vi "Get Ctr by Path.vi"() -> ()   [LabVIEW 2017]
uses:
  <vilib>/Utility/VariantDataType/VariantType.lvlib
panel:
  out "Value":variant
  out "Children":string
  in  "value":string="VI,127.0.0.1:3374,TC.vi/PNL_CTR,0/TAB_PAGE,0/PAGE_CTR,0/TAB_PAGE,10/PAGE_CTR,2"
  out "Cousins":string[](array[string])
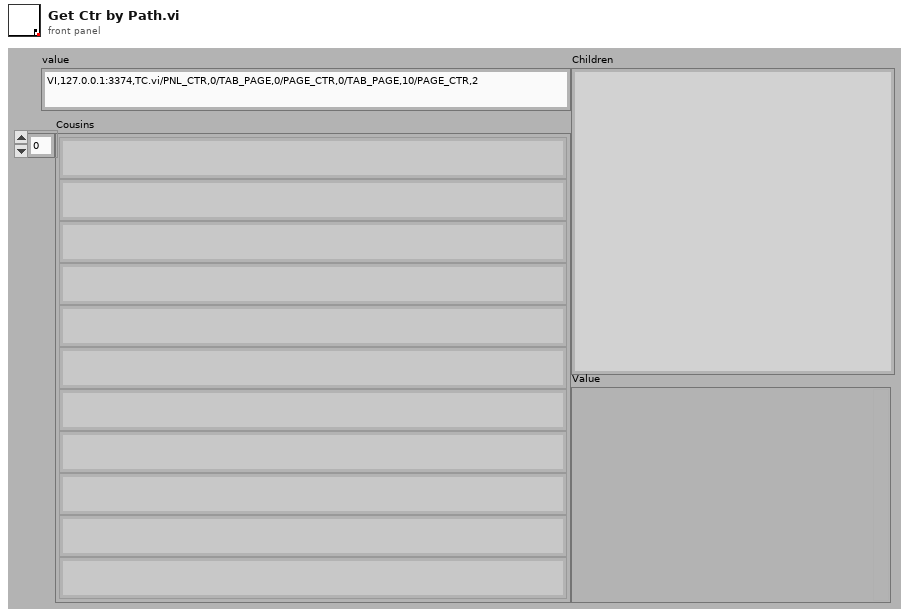
[diagram p1: front panel]
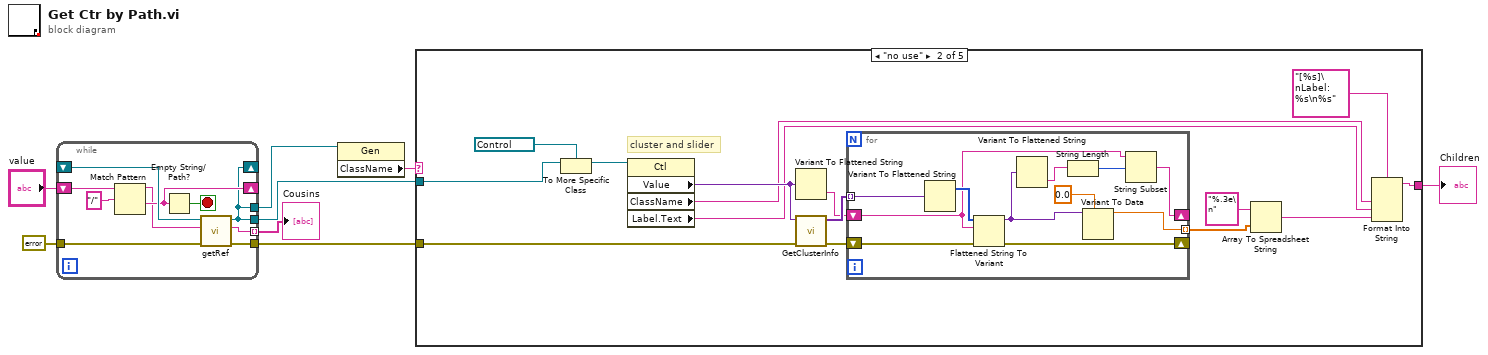
[diagram p0: block diagram]
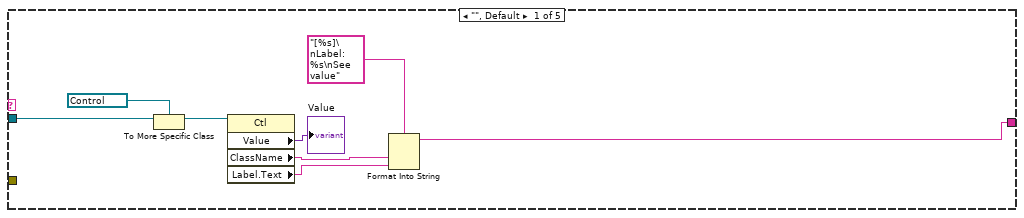
[diagram p2: hidden frame]
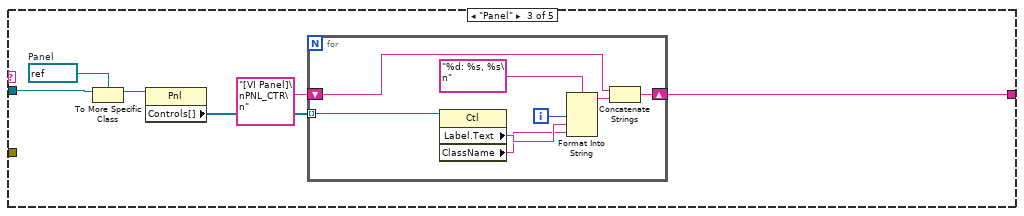
[diagram p3: hidden frame]
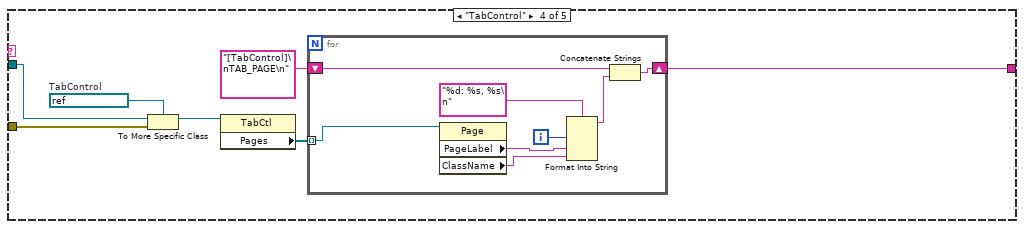
[diagram p4: hidden frame]
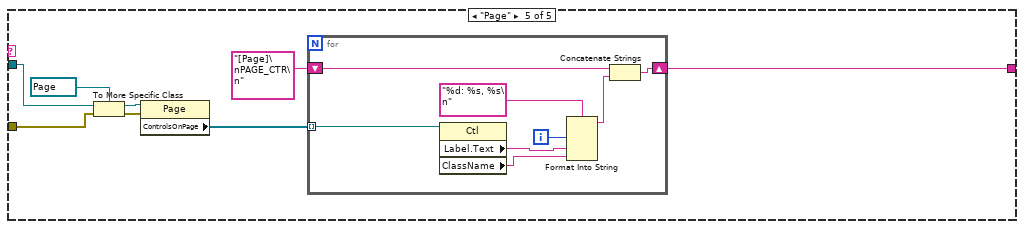
[diagram p5: hidden frame]
diagram:
  n1 = while {
    shift-right: [w14] -> _
    shift-left: "value" -> [w18]
    shift-right: [w9] -> _
    shift-left: _ -> [w15]
    tunnel: errorcluster {"status"=FALSE, "code"=0, "source"=""} ("error out") -> [w13]
    tunnel: [w12] -> w1
    tunnel: [w9] -> w8
    tunnel: [w10] -> w5 mode=indexing
    tunnel: [w9] -> w3
    stop <- w16 stop-if-true
    n2 = Match Pattern(string=w18, regular expression="/" ("搜索字符串/字符(-)")) -> (before substring=w11:string, after substring=w14:string)  [unwired: 3 out]
    n3 = Empty String/Path?(string/path=w14) -> (empty?=w16:bool)
    n4 = call "getRef.vi"("error in"=w13, "name"=w11, "Gen ref in"=w15) -> ("error out"=w12:errorcluster, "cousins"=w10:string, "Gen ref out"=w9:refnum<vi>)  [unwired: 6 out]
  }
  "Cousins" <- w5
  n5 = property class="Gen"(reference=w8) -> ("ClassName"=w4:string)  [unwired: 1 in, 2 out]
  n6 = case shown="\"no use\"" w4 {
    tunnel: w3 -> [w24 w39 w57 w72 w85]
    tunnel: [w22 w30 w53 w67 w82] -> w2
    tunnel: w1 -> [_ w37 _ w71 w86]
    frame "", Default {
      n7 = To More Specific Class(target class=refnum<vi> refnum ("引用"), reference=w24) -> (specific class reference=w26:refnum<vi>)  [unwired: 1 in, 1 out]
      n8 = property class="Ctl"(reference=w26) -> ("Value"=→"Value":variant, "ClassName"=w20:string, "Label.Text"=w19:string)  [unwired: 1 in, 2 out]
      n9 = Format Into String(format string="[%s]\nLabel: %s\nSee value", w20, w19) -> (resulting string=w22:string)  [unwired: 2 in, 1 out]
    }
    frame "no use" {
      # "cluster and slider"
      n10 = To More Specific Class(target class=refnum<vi> refnum ("引用"), reference=w39) -> (specific class reference=w41:refnum<vi>)  [unwired: 1 in, 1 out]
      n11 = property class="Ctl"(reference=w41) -> ("Value"=w38:variant, "ClassName"=w29:string, "Label.Text"=w28:string)  [unwired: 1 in, 2 out]
      n12 = Variant To Flattened String(Variant=w38) -> (data string=w35:string)  [unwired: 1 out]
      n13 = call <vilib>:"GetClusterInfo.vi"("error in (no error)"=w37, "Variant"=w38) -> ("error out"=w34:errorcluster, "Cluster Elements"=w36:variant[])  [unwired: 8 out]
      n14 = for {
        tunnel: w36 -> [w52] mode=indexing
        shift-right: [w47] -> _
        shift-left: w35 -> [w48]
        shift-right: [w45] -> _
        shift-left: w34 -> [w46]
        tunnel: [w42] -> w33 mode=indexing
        n15 = Variant To Flattened String(Variant=w52) -> (1:w51:i16[])  [unwired: 1 out]
        n16 = Flattened String To Variant(4:w46, 6:w48, 7:w51) -> (0:w45:errorcluster, 3:w44:variant)
        n17 = Variant To Flattened String(Variant=w44) -> (data string=w50:string)  [unwired: 1 out]
        n18 = String Length(string=w50) -> (length=w49:i32)
        n19 = Variant To Data(type=0.0, Variant=w44) -> (data=w42:dbl)  [unwired: 1 in, 1 out]
        n20 = String Subset(string=w48, offset (0)=w49) -> (substring=w47:string)  [unwired: 1 in]
      }
      n21 = Array To Spreadsheet String(array=w33, 3:"%.3e\n" ("format string")) -> (spreadsheet string=w27:string)  [unwired: 1 in]
      n22 = Format Into String(format string="[%s]\nLabel: %s\n%s", w29, w28, w27) -> (resulting string=w30:string)  [unwired: 2 in, 1 out]
    }
    frame "Panel" {
      w58 = refnum<vi> refnum  # Panel
      n23 = To More Specific Class(target class=w58, reference=w57) -> (specific class reference=w56:refnum<vi>)  [unwired: 1 in, 1 out]
      n24 = property class="Pnl"(reference=w56) -> ("Controls[]"=w55:refnum<vi>[])  [unwired: 1 in, 2 out]
      n25 = for {
        tunnel: w55 -> [w66] mode=indexing
        shift-right: [w61] -> w53
        shift-left: "[VI Panel]\nPNL_CTR\n" -> [w62]
        i -> [w65]
        n26 = property class="Ctl"(reference=w66) -> ("Label.Text"=w64:string, "ClassName"=w59:string)  [unwired: 1 in, 2 out]
        n27 = Format Into String(format string="%d: %s, %s\n", w65, w64, w59) -> (resulting string=w63:string)  [unwired: 2 in, 1 out]
        n28 = Concatenate Strings(w62, w63) -> (w61:string)
      }
    }
    frame "TabControl" {
      w73 = refnum<vi> refnum  # TabControl
      n29 = To More Specific Class(target class=w73, reference=w72, error in=w71) -> (specific class reference=w70:refnum<vi>)  [unwired: 1 out]
      n30 = property class="TabCtl"(reference=w70) -> ("Pages"=w69:refnum<vi>[])  [unwired: 1 in, 2 out]
      n31 = for {
        tunnel: w69 -> [w81] mode=indexing
        shift-right: [w77] -> w67
        shift-left: "[TabControl]\nTAB_PAGE\n" -> [w76]
        i -> [w80]
        n32 = property class="Page"(reference=w81) -> ("PageLabel"=w79:string, "ClassName"=w75:string)  [unwired: 1 in, 2 out]
        n33 = Format Into String(format string="%d: %s, %s\n", w80, w79, w75) -> (resulting string=w78:string)  [unwired: 2 in, 1 out]
        n34 = Concatenate Strings(w76, w78) -> (w77:string)
      }
    }
    frame "Page" {
      n35 = To More Specific Class(target class=refnum<vi> refnum ("元素"), reference=w85, error in=w86) -> (specific class reference=w88:refnum<vi>, error out=w89:errorcluster)
      n36 = property class="Page"(reference=w88, error in=w89) -> ("ControlsOnPage"=w84:refnum<vi>[])  [unwired: 2 out]
      n37 = for {
        tunnel: w84 -> [w97] mode=indexing
        shift-right: [w92] -> w82
        shift-left: "[Page]\nPAGE_CTR\n" -> [w93]
        i -> [w96]
        n38 = property class="Ctl"(reference=w97) -> ("Label.Text"=w95:string, "ClassName"=w91:string)  [unwired: 1 in, 2 out]
        n39 = Format Into String(format string="%d: %s, %s\n", w96, w95, w91) -> (resulting string=w94:string)  [unwired: 2 in, 1 out]
        n40 = Concatenate Strings(w93, w94) -> (w92:string)
      }
    }
  }
  "Children" <- w2
